vi "Toggle Switch.vi"(0 "On/Off Input":bool, 1 "START":bool=TRUE, 2 "Starting Value":bool, 3 "STOP":bool, 4 "On/Off Control":bool=TRUE, 5 "On Input":bool, 6 "On Control":bool=TRUE, 7 "Off Input":bool, 8 "Off Control":bool=TRUE, 9 "On Lock":bool, 10 "On Lock Control":bool=TRUE, 11 "Off Lock":bool, 12 "START CONTROL":bool=TRUE, 14 "STOP CONTROL":bool=TRUE, 15 "Off Lock Control":bool=TRUE) -> (13 "Output":bool)   [LabVIEW 2020]
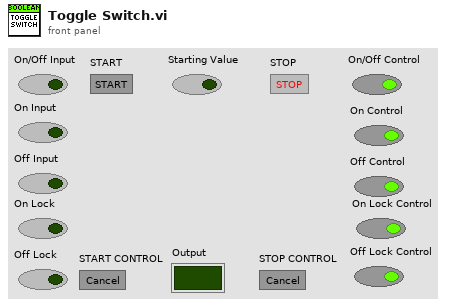
[diagram p1: front panel]
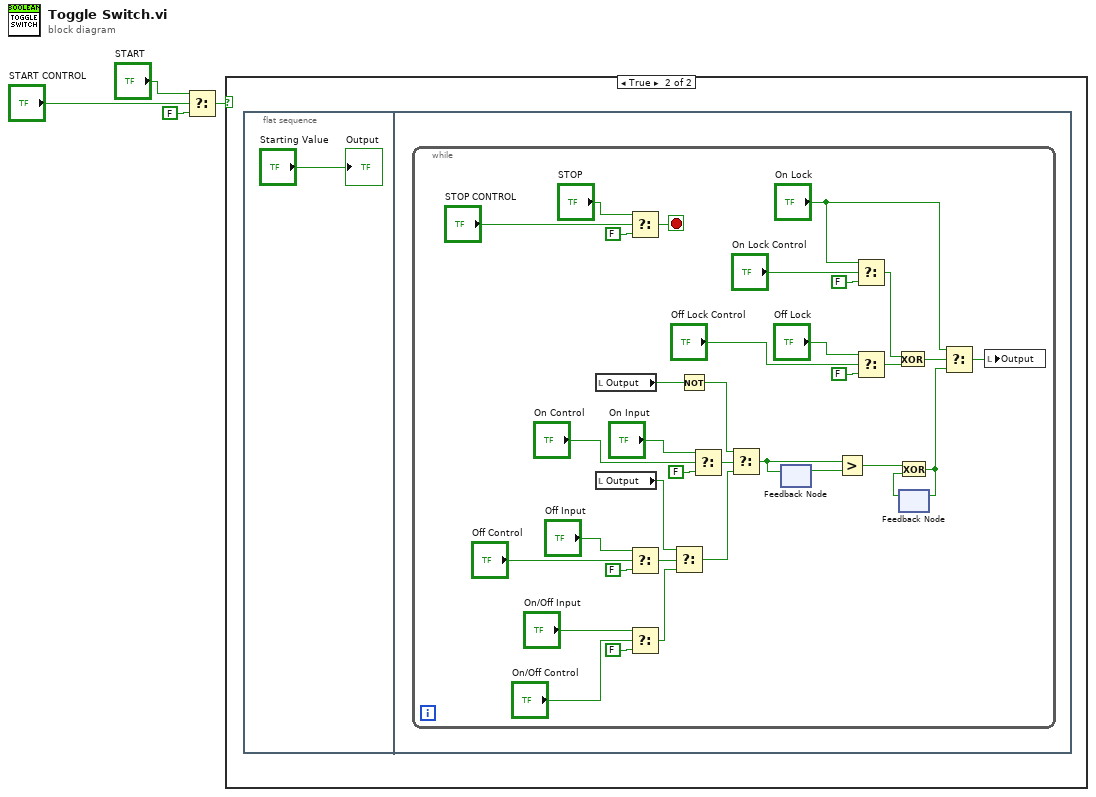
[diagram p0: block diagram]
diagram:
  n1 = Select(t="START", s="START CONTROL", f=FALSE) -> (s? t:f=w1:bool)
  n2 = case shown="True" w1 {
    frame False {
    }
    frame True {
      n3 = flat-sequence {
        frame #0 {
          "Output" <- "Starting Value"
        }
        frame #1 {
          n4 = while {
            stop <- w6 stop-if-true
            n5 = local read "Output"() -> (w27:bool)
            n6 = local read "Output"() -> (w28:bool)
            n7 = Select(t="STOP", s="STOP CONTROL", f=FALSE) -> (s? t:f=w6:bool)
            n8 = Select(t="Off Input", s="Off Control", f=FALSE) -> (s? t:f=w31:bool)
            n9 = Select(t="On/Off Input", s="On/Off Control", f=FALSE) -> (s? t:f=w22:bool)
            n10 = Select(t=w28, s=w31, f=w22) -> (s? t:f=w15:bool)
            n11 = Not(x=w27) -> (.not. x?=w26:bool)
            n12 = Select(t="On Input", s="On Control", f=FALSE) -> (s? t:f=w25:bool)
            n13 = Select(t=w26, s=w25, f=w15) -> (s? t:f=w17:bool)
            n14 = feedback #1() -> (w16:bool)  [unwired: 1 in]
            n15 = feedback-in #1(w17) -> ()
            n16 = Greater?(x=w17, y=w16) -> (0:w18:bool)
            n17 = Select(t="On Lock", s="On Lock Control", f=FALSE) -> (s? t:f=w35:bool)
            n18 = Select(t="Off Lock", s="Off Lock Control", f=FALSE) -> (s? t:f=w36:bool)
            n19 = Exclusive Or(1:w36, 2:w35) -> (0:w37:bool)
            n20 = feedback #2() -> (w19:bool)  [unwired: 1 in]
            n21 = Exclusive Or(1:w19, 2:w18) -> (0:w38:bool)
            n22 = feedback-in #2(w38) -> ()
            n23 = Select(t="On Lock", s=w37, f=w38) -> (s? t:f=w40:bool)
            n24 = local write "Output"(w40) -> ()
          }
        }
      }
    }
  }
